vi "Main (DAQ, SubVI, Tag).vi"() -> ()   [LabVIEW 2018]
doc: "Datenerfassung - Producer/Consumer mit Zustandsmaschine und Tag Channel\n\n* Analoges Eingangssigna, Definition des\nDAQmx Kanals im NI Max\n* Realisierung mit eine Zustandsmaschine\n* Drei Schleifen (Tasks): Zustandsmaschine und Datenerfassung und Auswertung\n*Realisierung des User Interfaces mit Event Structure\n* Kommunikation benutzereingaben (Zustandsmaschine) zu Datenerfassung mit \"Tag Channel\" und \"Stream Channel\"\n* Anzeige der Events\n* Anzeige der Zustände \"Messung/Warten/Auswertung\""
uses:
  Type Definitions/States UI.ctl
  Type Definitions/States Worker.ctl
  <extravilib>/ChannelInstances/Tag-t'States Worker.ctl'/Write With Abort.vi
  <extravilib>/ChannelInstances/Tag-t'States Worker.ctl'/Instantiate.vi
  <extravilib>/ChannelInstances/Tag-t'States Worker.ctl'/Endpoint.vi
  <extravilib>/ChannelInstances/Tag-t'States Worker.ctl'.lvlib
panel:
  in  "Tab Control":enum32{"Graph", "Average", "Chart"}(tab)=enum."Average"
  out "Graph":waveform(dbl)(graph)
  out "Average":waveform(dbl)(graph)
  out "Chart":waveform(dbl)(graph)
  out "Messung":bool
  out "Events":string="Exit= 1"
  in  "Messung":bool
  in  "Exit":bool
  out "Anzeige":dbl(knob) scale=4.5..5.5 scale format="%1.1f"
  # "Datenerfassung - \"UI/Worker\" mit Zustandsmaschine in SubVI und Tag Channel\n\n* Analoges Eingangssignal, Definition des\nDAQmx Kanals im NI Max\n*  Realisierung mit zwei Zustandsmaschi-nen (FSM)\n* Zustandsmaschine für UI Events und für Worker-Aufgabe\n* Zwei Schleifen (Tasks): UI und, Datenerfassung&Auswertung\n* Realisierung des User Interfaces mit Event Structure\n* Kommunikation Benutzereingaben (Zustandsmaschine) zu Datenerfassung mit \"Tag Channel\"\n\n* Anzeige der Events\n* Anzeige der Zustände \"Messung/Warten/Auswertung\"\n\n* Anzeige über \"Control References\" aus\nWorker VI in Main VI\n\nTiming:\n* Task 1Khz Sampling Rate und 100 Samples\n* Gemessen jede 0.1sec (continous\n\nFour Indicators\n* Gauge (filtered signal)\n* Graph (one scan)\n* Graph (sum of all scans)\n* Chart (all scans)"
  # "See below!"
  # "SubPanel display not possible!"
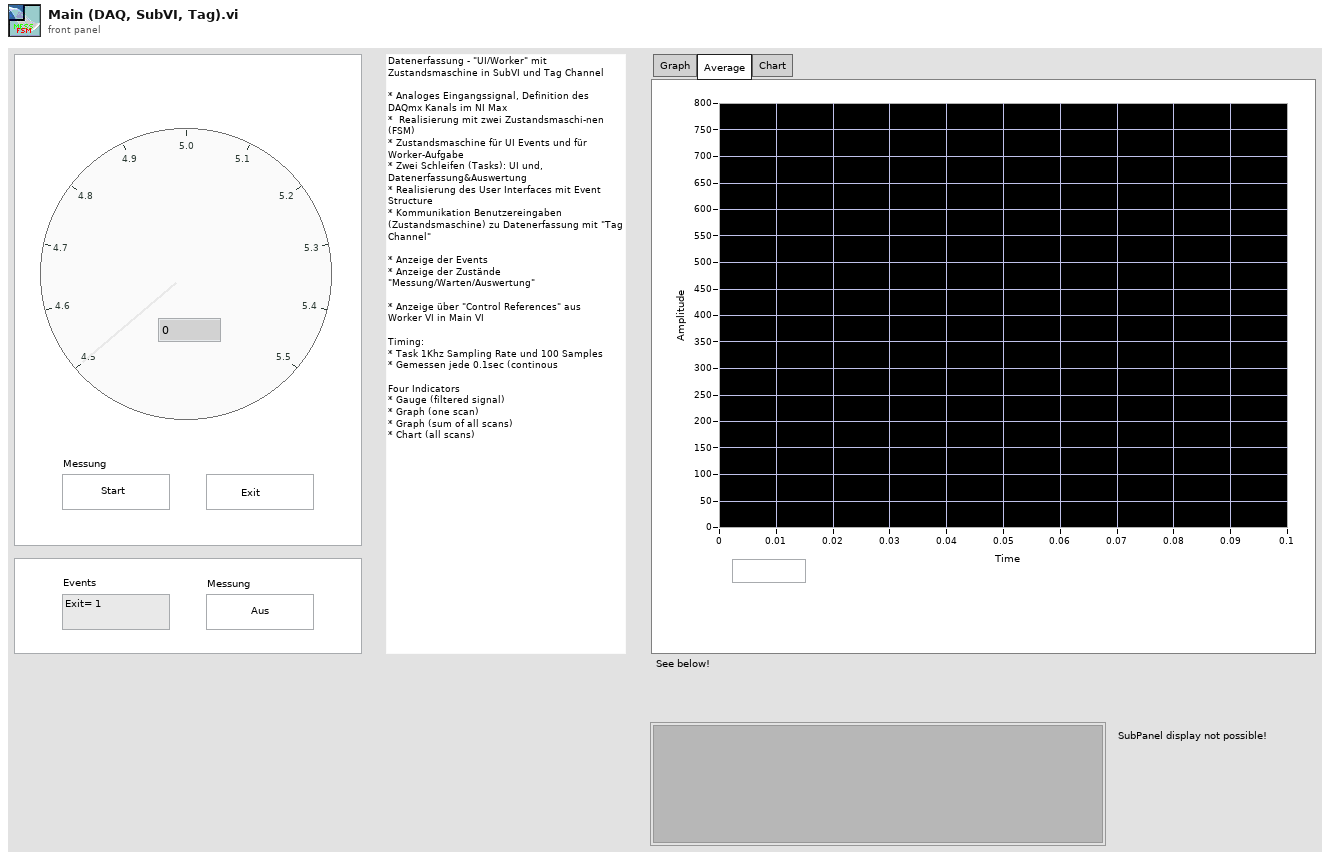
[diagram p1: front panel]
types:
  T1 = typedef "States UI.ctl" = enum16{"Initialize", "Wait for Event", "Exit"}
  T2 = typedef "States Worker.ctl" = enum16{"Messen", "Pausieren", "Exit"}
  T3 = typedef "Tag-t'States Worker.ctl'.lvlib/))Channel.ctl" = refnum<queue>
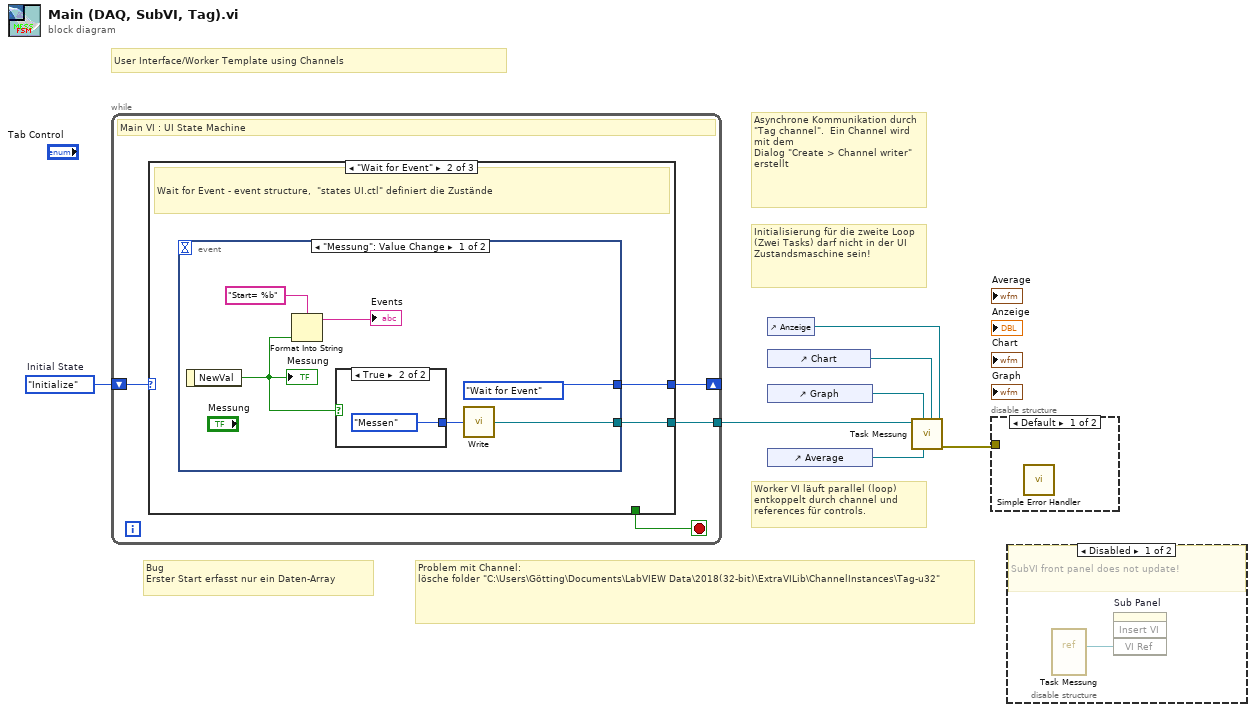
[diagram p0: block diagram]
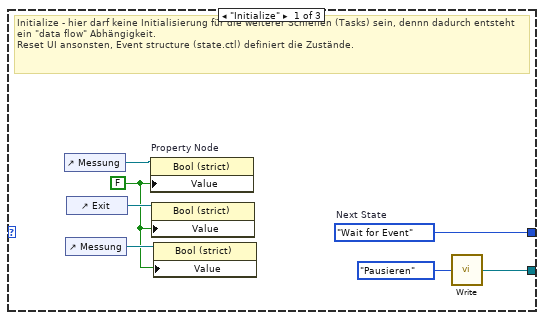
[diagram p3: hidden frame]
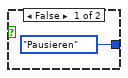
[diagram p4: hidden frame]
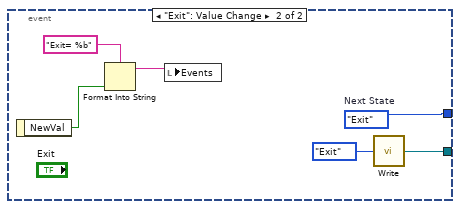
[diagram p5: hidden frame]
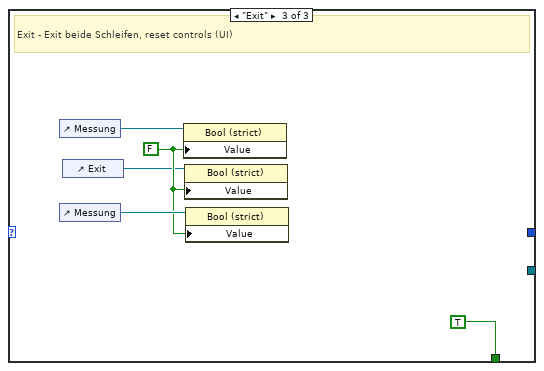
[diagram p6: hidden frame]
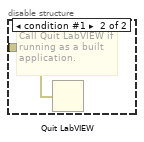
[diagram p7: hidden frame]
diagram:
  w7 = States_UI."Initialize"  # Initial State
  # "Worker VI läuft parallel (loop)\nentkoppelt durch channel und\nreferences für controls."
  # "Bug\nErster Start erfasst nur ein Daten-Array"
  # "User Interface/Worker Template using Channels"
  # "Problem mit Channel:\nlösche folder \"C:\\Users\\Götting\\Documents\\LabVIEW Data\\2018(32-bit)\\ExtraVILib\\ChannelInstances\\Tag-u32\""
  # "Initialisierung für die zweite Loop (Zwei Tasks) darf nicht in der UI Zustandsmaschine sein!"
  # "Asynchrone Kommunikation durch\n\"Tag channel\".  Ein Channel wird mit dem\nDialog \"Create > Channel writer\" erstellt"
  n1 = while {
    shift-right: [w10] -> _
    shift-left: w7 -> [w11]
    tunnel: [w8] -> w3
    stop <- w9 stop-if-true
    # "Main VI : UI State Machine"
    n2 = case shown="\"Wait for Event\"" w11 {
      tunnel: [w18 w20 _] -> w10
      tunnel: [_ _ TRUE ("Stop Loop?")] -> w9
      tunnel: [w12 w19 _] -> w8
      frame "Initialize" {
        w14 = FALSE ("Value")
        w18 = States_UI."Wait for Event"  # Next State
        # "Initialize - hier darf keine Initialisierung für die weiterer Schleifen (Tasks) sein, dennn dadurch entsteht ein \"data flow\" Abhängigkeit. \nReset UI ansonsten, Event structure (state.ctl) definiert die Zustände."
        n3 = control-ref of="Messung"() -> (w17:refnum<vi>)
        n4 = control-ref of="Messung"() -> (w15:refnum<vi>)
        n5 = control-ref of="Exit"() -> (w16:refnum<vi>)
        n6 = property on="Property Node" class="Bool (strict)"(reference=w17, "Value"=w14) -> ()  [unwired: 1 in, 2 out]
        n7 = property class="Bool (strict)"(reference=w16, "Value"=w14) -> ()  [unwired: 1 in, 2 out]
        n8 = property class="Bool (strict)"(reference=w15, "Value"=w14) -> ()  [unwired: 1 in, 2 out]
        n9 = call <extravilib>:"Write.vi"("element"=States_Worker."Pausieren" ("States")) -> ("channel"=w12:T3)  [unwired: 1 out]
      }
      frame "Wait for Event" {
        # "Wait for Event - event structure,  \"states UI.ctl\" definiert die Zustände"
        n10 = event shown="[0] \"Messung\": Value Change" {
          selector: _ -> [_ _]
          dyn-events: _ -> [_ _]
          timeout: _ -> [_ _]
          tunnel: [States_UI."Wait for Event" ("Next State") w34] -> w20
          tunnel: [w21 w29] -> w19
          event "Messung": Value Change {
            n11 = event-data() -> ("NewVal"=w23:bool)  [unwired: 1 in]
            "Messung" <- w23
            n12 = Format Into String(format string="Start= %b", w23) -> (resulting string=→"Events":string)  [unwired: 2 in, 1 out]
            n13 = case shown="True" w23 {
              tunnel: [States_Worker."Pausieren" ("Initial State") States_Worker."Messen" ("Initial State")] -> w22
              frame False {
              }
              frame True {
              }
            }
            n14 = call <extravilib>:"Write.vi"("element"=w22) -> ("channel"=w21:T3)  [unwired: 1 out]
          }
          event "Exit": Value Change {
            w34 = States_UI."Exit"  # Next State
            n15 = event-data() -> ("NewVal"=w32:bool)  [unwired: 1 in]
            n16 = Format Into String(format string="Exit= %b", w32) -> (resulting string=w33:string)  [unwired: 2 in, 1 out]
            n17 = local write "Events"(w33) -> ()
            n18 = call <extravilib>:"Write.vi"("element"=States_Worker."Exit" ("States")) -> ("channel"=w29:T3)  [unwired: 1 out]
          }
        }
      }
      frame "Exit" {
        w37 = FALSE ("Value")
        # "Exit - Exit beide Schleifen, reset controls (UI)"
        n19 = control-ref of="Messung"() -> (w39:refnum<vi>)
        n20 = control-ref of="Messung"() -> (w38:refnum<vi>)
        n21 = control-ref of="Exit"() -> (w36:refnum<vi>)
        n22 = property class="Bool (strict)"(reference=w39, "Value"=w37) -> ()  [unwired: 1 in, 2 out]
        n23 = property class="Bool (strict)"(reference=w36, "Value"=w37) -> ()  [unwired: 1 in, 2 out]
        n24 = property class="Bool (strict)"(reference=w38, "Value"=w37) -> ()  [unwired: 1 in, 2 out]
      }
    }
  }
  n25 = control-ref of="Anzeige"() -> (w4:refnum<vi>)
  n26 = control-ref of="Chart"() -> (w6:refnum<vi>)
  n27 = control-ref of="Graph"() -> (w5:refnum<vi>)
  n28 = control-ref of="Average"() -> (w2:refnum<vi>)
  n29 = call "Task Messung.vi"("Gauge"=w4, "Chart"=w6, "Average"=w2, "Graph"=w5, "Channel in"=w3) -> ("error out"=w1:errorcluster)  [unwired: 6 in]
  n30 = disable-structure shown="Default" {
    disable-tunnel: w1 -> [_ w40]
    frame condition #0 (active) {
      n31 = call <vilib>:"Simple Error Handler.vi"() -> ()  [unwired: 5 in, 5 out]
    }
    frame condition #1 {
      # "Call Quit LabVIEW if running as a built application."
      n32 = Quit LabVIEW(quit? (T)=w40) -> ()
    }
  }
  n33 = disable-structure shown="Disabled" {
    frame Disabled {
      # "SubVI front panel does not update!"
      n34 = vi-ref "Task Messung.vi"() -> (w41:refnum<vi>)
      n35 = invoke on="Sub Panel" class="SubPnl" method="Insert VI"("VI Ref"=w41) -> ()  [unwired: 3 in, 4 out]
    }
    frame Enabled {
    }
  }
